vi "Send Command.vi"(3 "BCI-1553 Device":refnum<k21>, 4 "Data 3":u16, 5 "BCI-1553-RSP":refnum<k21>, 6 "Data 2":u16, 7 "Target ID":u8, 8 "Data 1":u16, 10 "Command":u8) -> ()   [LabVIEW 2020, in "BCI-1553 RT Interface.lvlib"]
doc: "Sends a command to a module."
uses:
  BCI-1553 RT Interface.lvlib
  <vilib>/rvi/eio/common/nirviEmuTemplateMethod_errors.vi
  <vilib>/rvi/DataTransferAndStorage/Container/Common/niFpgaContainerExecOnDevCompGetState.vi
  <vilib>/rvi/Emulation/niFpgaEmulationIsFPGAContextNoSignature.vi
  <vilib>/rvi/Emulation/niFpgaSctlEmulationGetInTimedLoop.vi
  <vilib>/rvi/errors/niFpgaSetErrorForExecOnDevCompSimple.vi
  <vilib>/rvi/eio/common/nirviEmuReportErrorAndStop.vi
  <vilib>/rvi/DataTransferAndStorage/Container/Common/niFpgaContainerGetUniqueNameForEmu.vi
  <vilib>/rvi/FIFO/Fifo_Resource/nirvififoEmulationSetSize.vi
  <vilib>/rvi/FIFO/Fifo_Resource/nirviFifoEmulationQueueMgr.vi
  <instcachedir>/0/nirviFifoEmulationQueueMgr_E5CAEC123FF24DC58D834DCA3CDAA9B5.lvgen/nirviFifoEmulationQueueMgr_E5CAEC123FF24DC58D834DCA3CDAA9B5_001.vi
  <vilib>/rvi/FIFO/Fifo_Resource/nirvififoEmulationDetermineInputValidOut.vi
  <vilib>/rvi/FIFO/Fifo_Resource/nirvififoEmulationCreateLock.vi
  <vilib>/rvi/Emulation/niFpgaProcessEmulError.vi
  <vilib>/rvi/FIFO/Fifo_Resource/nirvififoEmulationObtainLock.vi
  <vilib>/rvi/FIFO/Fifo_Resource/nirvififoEmulationReleaseLock.vi
  <vilib>/rvi/occurrence/nirviWaitOnOccurrenceBase.vi
  <vilib>/rvi/errors/nirviReportUnexpectedCaseInternalError.vi
  <vilib>/rvi/errors/nirviReportUnexpectedCaseInternalError (U32).vi
  <vilib>/Utility/error.llb/Clear Errors.vi
  <vilib>/rvi/interface/RandomDataEmulation/niFpgaRandomDataHandleErrors.vi
  <vilib>/eio/EIOMethodNode/EIOMethodNode.xnode
  <vilib>/rvi/DataTransferAndStorage/Container/XNode/niFpgaContainer.xnode
  <vilib>/rvi/FIFO/Fifo_Resource/niFpgaFifoEmulationRefIn.vi
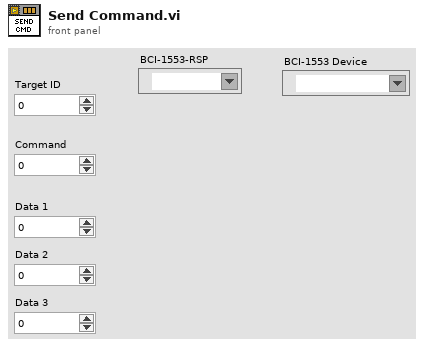
[diagram p1: front panel]
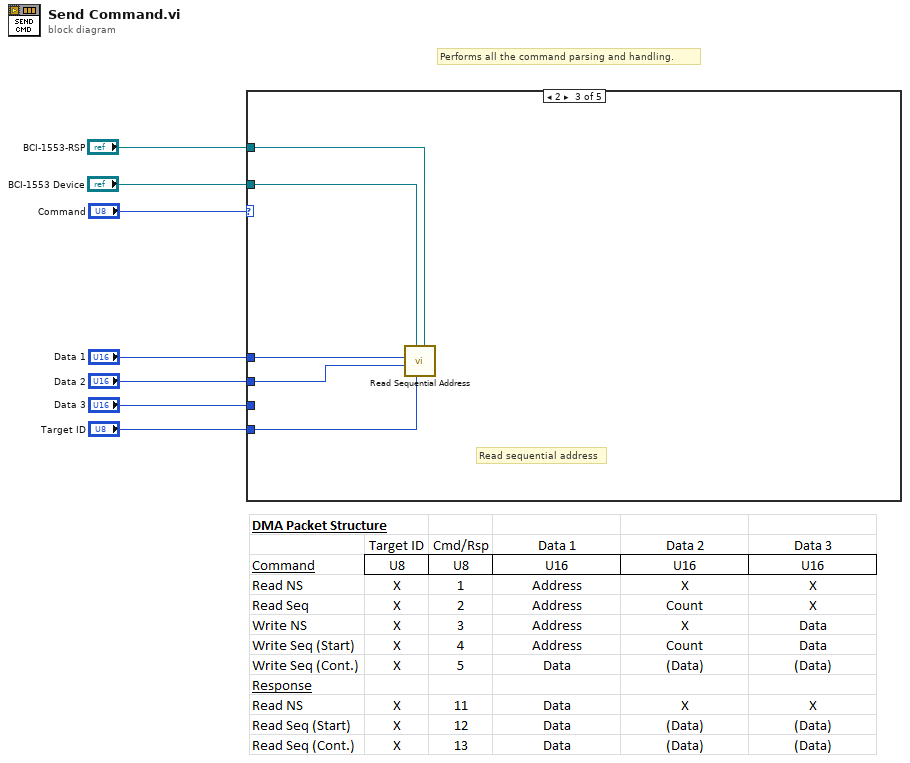
[diagram p0: block diagram]
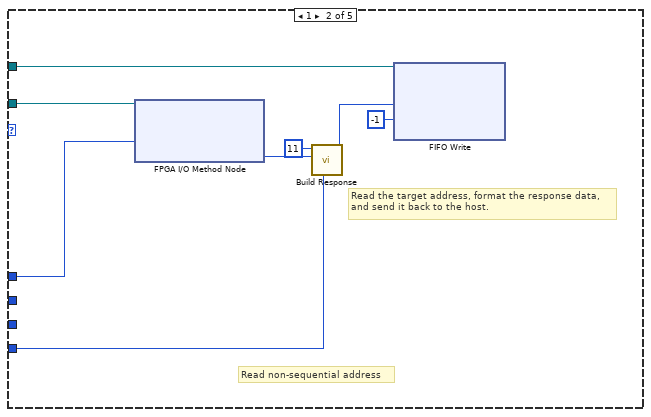
[diagram p3: hidden frame]
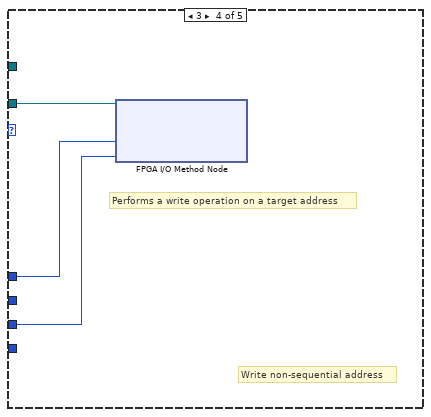
[diagram p4: hidden frame]
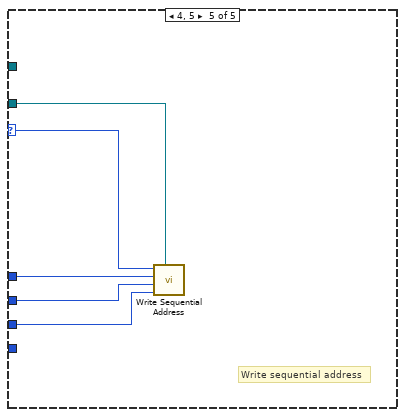
[diagram p5: hidden frame]
diagram:
  # "Performs all the command parsing and handling."
  n1 = case shown="2" "Command" {
    selector: "Command" -> [_ _ _ _ w27]
    tunnel: "Data 1" -> [_ w14 w18 w22 w26]
    tunnel: "Data 2" -> [_ _ w17 _ w25]
    tunnel: "Data 3" -> [_ _ _ w21 w24]
    tunnel: "BCI-1553-RSP" -> [_ w13 w19 _ _]
    tunnel: "BCI-1553 Device" -> [_ w15 w20 w23 w28]
    tunnel: "Target ID" -> [_ w8 w16 _ _]
    frame 0, Default {
      # "Do nothing when we receive an unsupported command."
    }
    frame 1 {
      # "Read the target address, format the response data,\nand send it back to the host."
      # "Read non-sequential address"
      n2 = xnode "FPGA I/O Method Node"("FPGA I/O In"=w15, "Address"=w14) -> ("Data"=w11:u16)  [unwired: 1 out]
      n3 = call "Build Response.vi"("Target ID"=w8, "Data 1"=w11, "Response"=u8 11) -> ("Response Value"=w10:u64)  [unwired: 8 in]
      n4 = xnode "FIFO Write"("Element"=w10, "Timeout"=-1, "FIFO In"=w13) -> ()  [unwired: 2 out]
    }
    frame 2 {
      # "Read sequential address"
      n5 = call "Read Sequential Address.vi"("BCI-1553-RSP"=w19, "Target ID"=w16, "BCI-1553 Device"=w20, "Count"=w17, "Address"=w18) -> ()  [unwired: 7 in]
    }
    frame 3 {
      # "Performs a write operation on a target address"
      # "Write non-sequential address"
      n6 = xnode "FPGA I/O Method Node"("FPGA I/O In"=w23, "Address"=w22, "Data"=w21) -> ()  [unwired: 1 out]
    }
    frame 4, 5 {
      # "Write sequential address"
      n7 = call "Write Sequential Address.vi"("BCI-1553 Device"=w28, "Data 3"=w24, "Data 2"=w25, "Data 1"=w26, "Command"=w27) -> ()  [unwired: 7 in]
    }
  }
